vi "LabVIEW JSON VI Tree.vi"   [LabVIEW 2019]
doc: "LabVIEW JSON VI Tree\nCreated by: Ryan Pacini"
uses:
  lib/Element.ctl
  lib/Element Type.ctl
  lib/Element Set Behavior.ctl
  lib/labview_json.lvlib
types:
  T1 = typedef "labview_json.lvlib/Element Set Behavior.ctl" = enum8{"Add or Modify", "Modify Only", "Replace"}
  T2 = typedef "labview_json.lvlib/Element.ctl" = cluster{"Key":string, "Type":T3, "Value":variant, "IsRootPath":bool}
  T3 = typedef "labview_json.lvlib/Element Type.ctl" = enum8{"NULL", "OBJECT", "ARRAY", "BOOL", "INT", "UINT", "FLOAT", "STRING"}
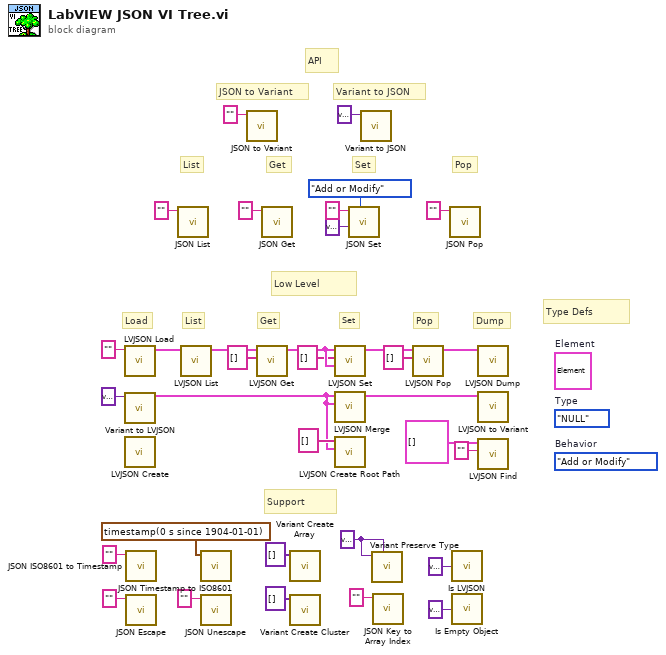
[diagram p0: block diagram]
diagram:
  w13 = variant ("Variant in")
  (unwired) Element_Set_Behavior."Add or Modify"  # Behavior
  (unwired) T2 {"Key"="", "Type"=enum."NULL", "Value"=variant, "IsRootPath"=FALSE}  # Element
  (unwired) Element_Type."NULL"  # Type
  # "Type Defs"
  # "Support"
  # "Low Level"
  # "API"
  # "Pop"
  # "Set"
  # "Get"
  # "List"
  # "Pop"
  # "Variant to JSON"
  # "JSON to Variant"
  # "Set"
  # "Get"
  # "List"
  # "Dump"
  # "Load"
  n1 = call "LVJSON Load.vi"("JSON in"="") -> ("Root Element out"=w25:T2)  [unwired: 9 in, 1 out]
  n2 = call "Variant to LVJSON.vi"("Variant in"=variant) -> ("Element out"=w4:T2)  [unwired: 9 in, 1 out]
  n3 = call "LVJSON Create.vi"() -> ()  [unwired: 11 in, 1 out]
  n4 = call "JSON ISO8601 to Timestamp.vi"("ISO 8601 Date Time"="") -> ()  [unwired: 10 in, 1 out]
  n5 = call "JSON Escape.vi"("String"="") -> ()  [unwired: 9 in, 2 out]
  n6 = call "JSON List.vi"("JSON in"="") -> ()  [unwired: 7 in, 4 out]
  n7 = call "LVJSON List.vi"("Root Element in"=w25) -> ("dup Root Element"=w24:T2)  [unwired: 7 in, 3 out]
  n8 = call "JSON Timestamp to ISO8601.vi"("Local Date Time"=timestamp(0 s since 1904-01-01)) -> ()  [unwired: 10 in, 1 out]
  n9 = call "JSON Unescape.vi"("Escaped String"="") -> ()  [unwired: 9 in, 2 out]
  n10 = call "JSON to Variant.vi"("JSON"="") -> ()  [unwired: 9 in, 2 out]
  n11 = call "LVJSON Get.vi"("Root Path"=string[] [], "Root Element in"=w24) -> ("dup Root Element"=w5:T2)  [unwired: 6 in, 3 out]
  n12 = call "JSON Get.vi"("JSON in"="") -> ()  [unwired: 8 in, 3 out]
  n13 = call "Variant Create Array.vi"("Elements"=variant[] []) -> ()  [unwired: 9 in, 2 out]
  n14 = call "Variant Create Cluster.vi"("Elements"=variant[] []) -> ()  [unwired: 9 in, 2 out]
  n15 = call "LVJSON Set.vi"("Element"=w5, "Root Path"=string[] [], "Root Element in"=w5) -> ("Root Element out"=w23:T2)  [unwired: 6 in, 2 out]
  n16 = call "LVJSON Merge.vi"("Element to Merge"=w4, "Root Element in"=w4) -> ("Root Element out"=w7:T2)  [unwired: 7 in, 2 out]
  n17 = call "LVJSON Create Root Path.vi"("Element in"=w4, "Root Path"=string[] []) -> ()  [unwired: 8 in, 2 out]
  n18 = call "JSON Set.vi"("Behavior (Add or Modify)"=Element_Set_Behavior."Add or Modify", "Value"=variant, "JSON in"="") -> ()  [unwired: 6 in, 3 out]
  n19 = call "Variant to JSON.vi"("Variant in"=variant) -> ()  [unwired: 9 in, 2 out]
  n20 = call "Variant Preserve Type.vi"("Variant Type"=w13, "Variant in"=w13) -> ()  [unwired: 8 in, 2 out]
  n21 = call "JSON Key to Array Index.vi"("Key"="") -> ()  [unwired: 8 in, 3 out]
  n22 = call "LVJSON Pop.vi"("Root Path"=string[] [], "Root Element in"=w23) -> ("Root Element out"=w22:T2)  [unwired: 6 in, 3 out]
  n23 = call "JSON Pop.vi"("JSON in"="") -> ()  [unwired: 7 in, 4 out]
  n24 = call "Is LVJSON.vi"("Variant"=variant) -> ()  [unwired: 1 out]
  n25 = call "Is Empty Object.vi"("Variant"=variant) -> ()  [unwired: 1 out]
  n26 = call "LVJSON Dump.vi"("Root Element in"=w22) -> ()  [unwired: 8 in, 3 out]
  n27 = call "LVJSON to Variant.vi"("Root Element in"=w7) -> ()  [unwired: 8 in, 3 out]
  n28 = call "LVJSON Find.vi"("Key"="", "Elements in"=T2[] []) -> ()  [unwired: 8 in, 2 out]
